vi "Get Calproc.vi"(7 "제목":refnum<vi>, 8 "에러 입력":errorcluster caption="에러 입력(에러 없음)", 11 "Func_ext":string) -> (0 "에러 출력":errorcluster, 1 "Condition":string[][](array[string]), 3 "Func_ext Out":string, 6 "클러스터":T1)   [LabVIEW 2020]
uses:
  Controls/Clst_Get Calproc.ctl
  Controls/Cmd_Read Query.ctl
  Controls/Clst_Query Info.ctl
  Controls/Cmd_File path.ctl
  Controls/Cmd_File Type.ctl
  Variables/Global_Cal Info.vi
  Public/Polymorph/Data Class_2D Str.vi
  Public/Polymorph/Rmv Empt Arr_2D Str.vi
  <vilib>/Utility/file.llb/Read Delimited Spreadsheet (string).vi
  Public/Polymorph/Array Dedup_2D Str.vi
  <vilib>/addons/database/NI_Database_API.lvlib
panel:
  out "제목":string
  out "Data 2":string[][](array[string])
  out "Data":string[][](array[string])
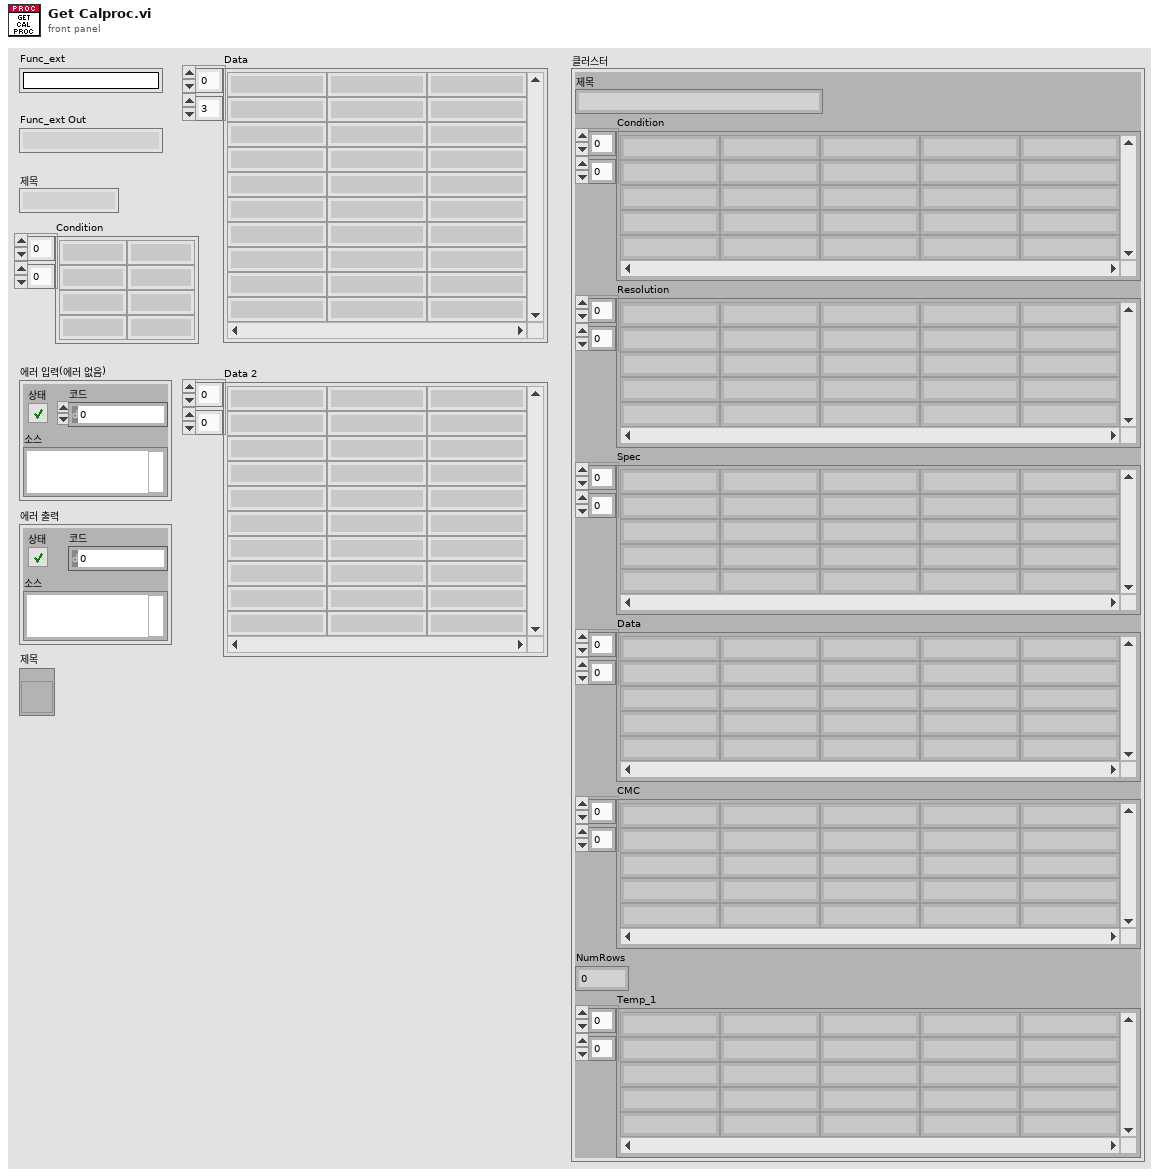
[diagram p1: front panel]
types:
  T1 = typedef "Clst_Get Calproc.ctl" = cluster{"제목":string, "Condition":string[][], "Resolution":string[][], "Spec":string[][], "Data":string[][], "CMC":string[][], "NumRows":u32, "Temp_1":string[][]}
  T2 = typedef "Cmd_Read Query.ctl" = enum16{"교정자 이름 얻기", "인증교정자 얻기", "기술책임자 얻기", "기책부책 얻기", "등록번호 얻기", "등록정보 얻기", "업체정보 얻기", "교정일자(CAMAS) 얻기", "교정일자(CALSTD) 얻기", "교정환경 얻기", "교정절차서 목록 얻기", "교정절차서명 얻기", "교정절차 목록얻기", "교정절차 얻기", "PROC 교정절차 얻기", "PROC SPEC 얻기", "교정절차(Func별) 얻기", "교정절차(Func_ext별) 얻기", "기관코드 얻기", "교정기능(세부분류) 얻기", "교정기능(모델) 얻기", "교정기능 목록 얻기", "교정기능 명칭 얻기", "교정기능 항목명칭 얻기", "DB (사용기준기) 얻기", "DB (기준기이름) 얻기", "DB (기준기이름목록) 얻기", "DB (기준기목록) 얻기", "DB (기준기값) 얻기", "DB (CMC) 얻기", "DB (FUNC) 얻기", "DB (CALNAME) 얻기", "DB (STDNAME) 얻기", "DB (SPEC) 얻기", "모델(항목전체) 얻기", "모델(최대범위) 얻기", "모델(최소범위) 얻기", "모델(최대최소) 얻기", "모델(범위조건) 얻기", "모델(등록요청) 얻기", "모델(형식별) 얻기", "모델(조건별) 얻기", "모델(모델검색) 얻기", "세부분류 목록 얻기", "기준기등록리스트 얻기", "STD Cal Date Check", "DB등록일자 얻기", "적용항목 얻기", "기타정보 얻기", "기준기요청 얻기", "서버버전 얻기"}
  T3 = typedef "Clst_Query Info.ctl" = cluster{"사번":string, "등록번호":string, "업체명":string, "세부분류코드":string, "형식":string, "기기번호":string, "FUNC":string, "FUNC_EXT":string, "옵션":string, "추가문자열":string, "일자":string, "배열 1":string[], "배열 2":string[], "항목명":string, "문자열":string, "이름":string}
  T4 = cluster{"세부분류코드":string, "형식":string, "옵션":string, "측정기명":string, "EXCEL파일명":string, "TEMP":string}
  T5 = typedef "NI_Database_API.lvlib/Conn ObjectReference.ctl" = refnum<k1>
  T6 = typedef "Cmd_File Type.ctl" = enum16{"엑셀", "엑셀(2003)", "텍스트", "설정", "2진", "VI", "CSV", "LOG", "폴더"}
  T7 = typedef "Cmd_File path.ctl" = enum16{"에러로그", "데이터파일경로", "성적서원본", "지난성적서", "Data Files", "경로생성", "Updater", "Template", "설정파일경로", "FTP Upload", "Update 경로", "어플리케이션"}
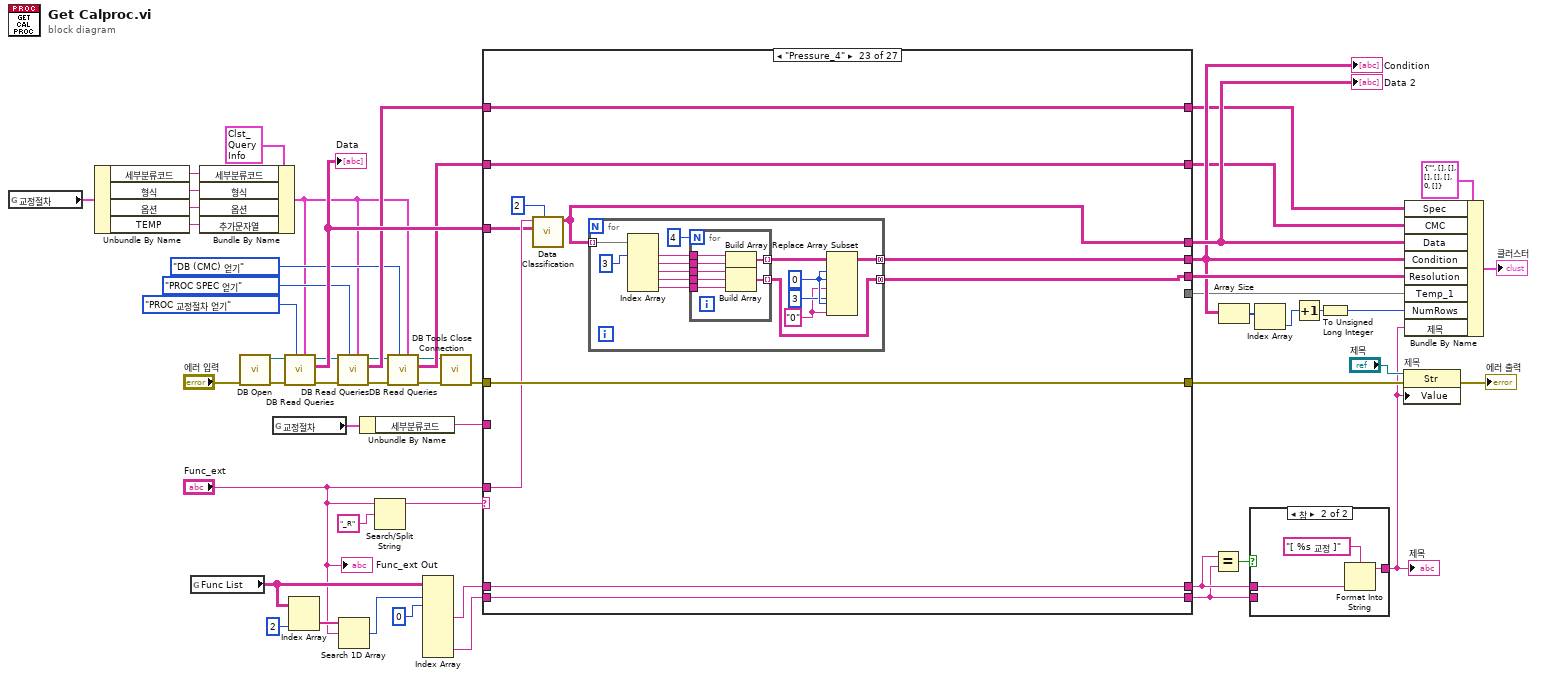
[diagram p0: block diagram]
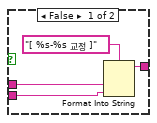
[diagram p2: hidden frame]
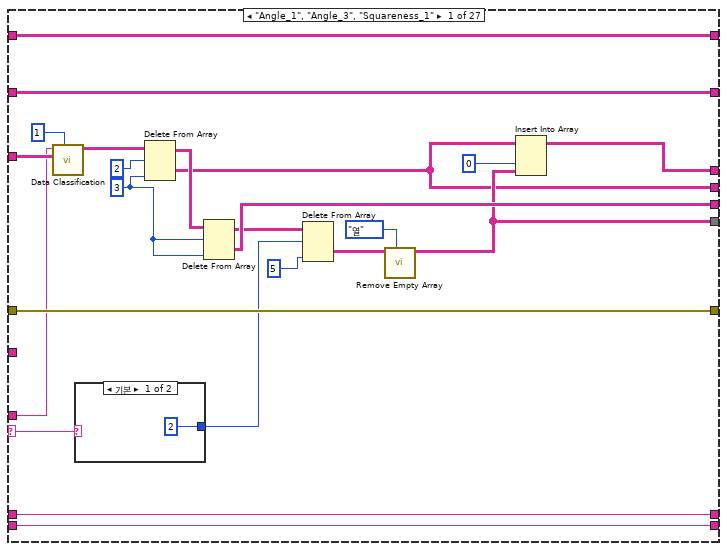
[diagram p3: hidden frame]
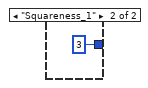
[diagram p4: hidden frame]
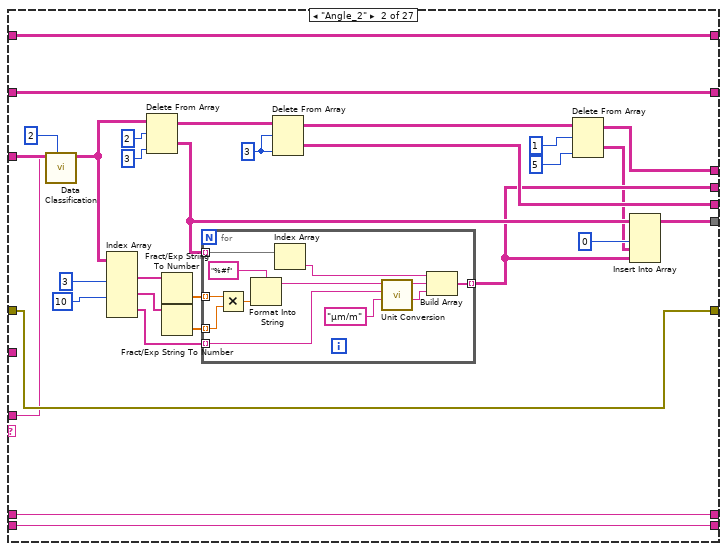
[diagram p5: hidden frame]
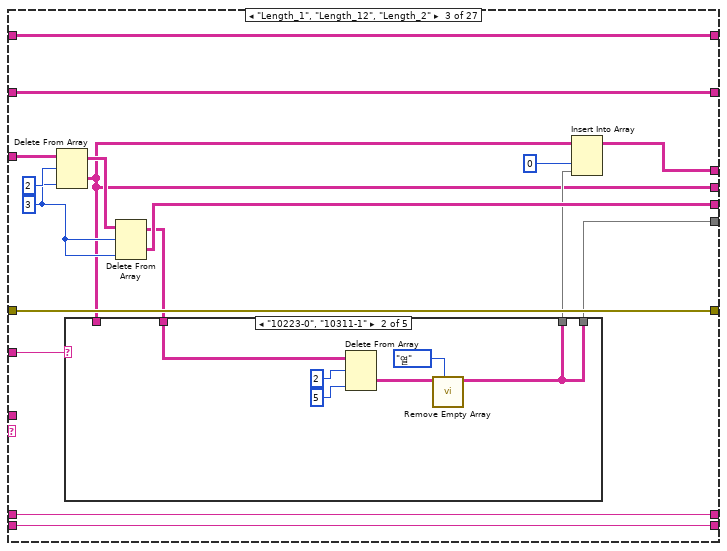
[diagram p6: hidden frame]
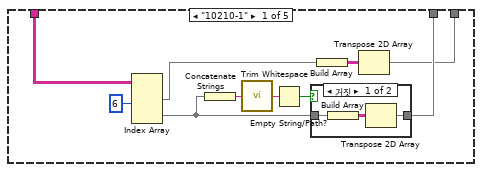
[diagram p7: hidden frame]
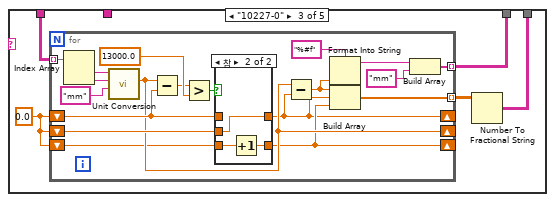
[diagram p9: hidden frame]
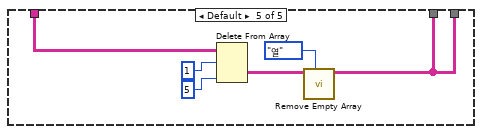
[diagram p12: hidden frame]
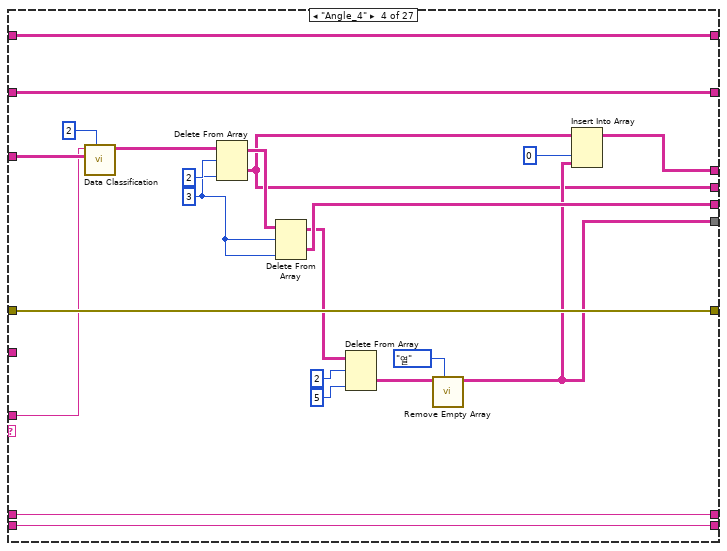
[diagram p13: hidden frame]
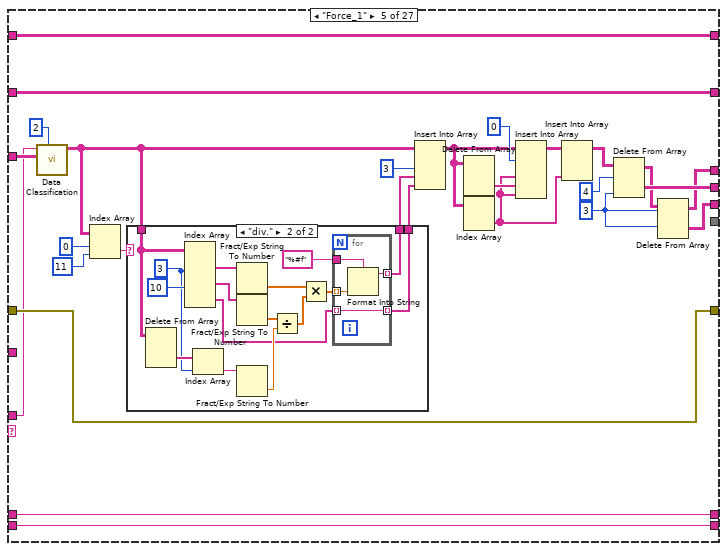
[diagram p14: hidden frame]
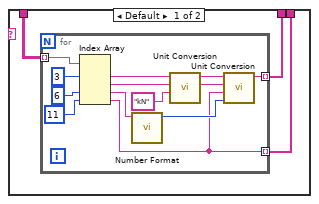
[diagram p15: hidden frame]
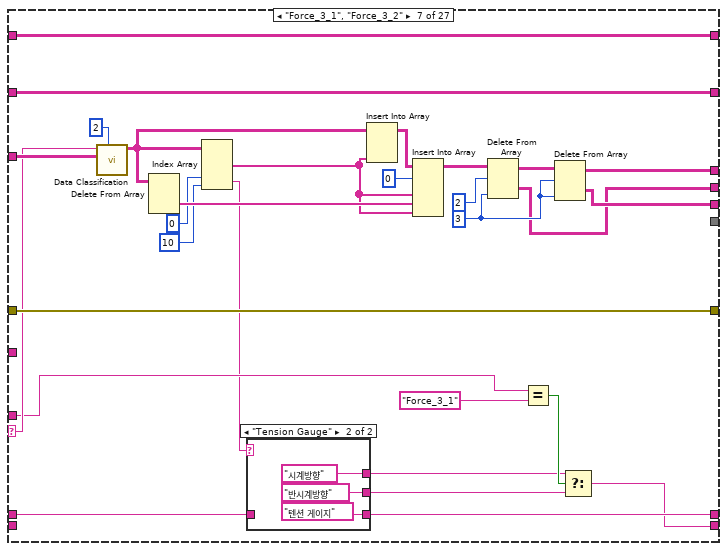
[diagram p17: hidden frame]
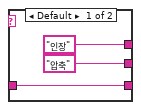
[diagram p18: hidden frame]
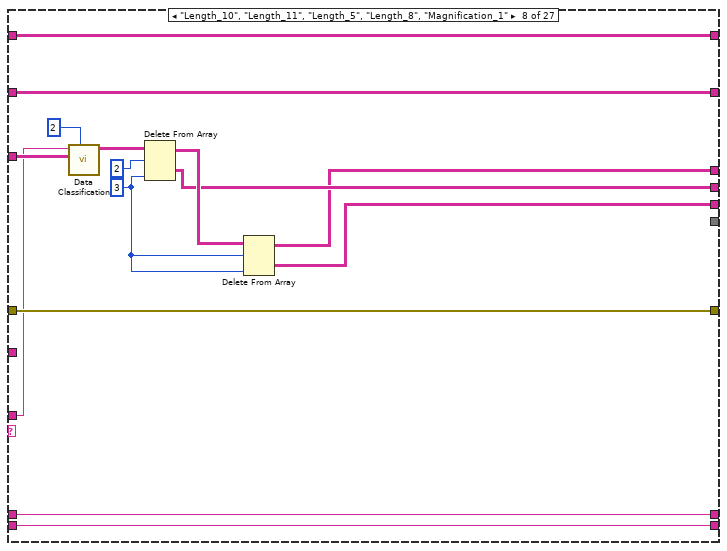
[diagram p19: hidden frame]
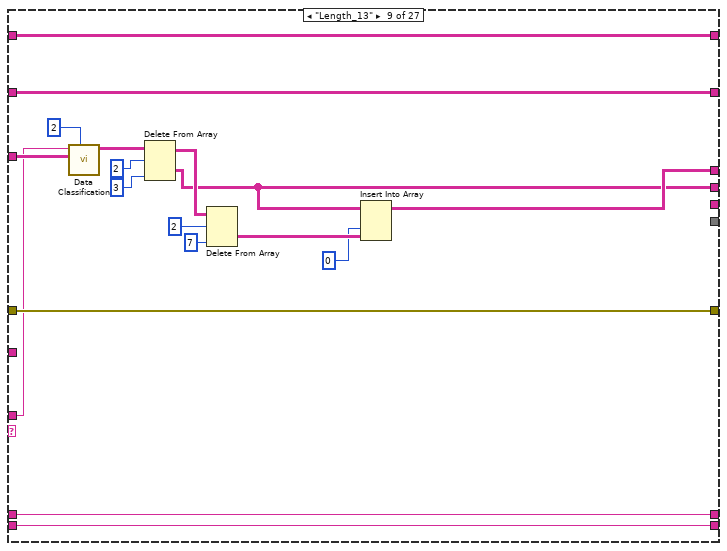
[diagram p20: hidden frame]
diagram:
  n1 = global read "Global_Cal Info.vi" "교정절차"() -> (w29:T4)
  n2 = Unbundle By Name(w29) -> ("세부분류코드"=w28:string, "형식"=w27:string, "옵션"=w26:string, "TEMP"=w13:string)
  n3 = global read "Global_Cal Info.vi" "Func List"() -> (w39:string[][])
  n4 = Bundle By Name(cluster=T3 {"사번"="", "등록번호"="", "업체명"="", "세부분류코드"="", "형식"="", "기기번호"="", "FUNC"="", "FUNC_EXT"="", "옵션"="", "추가문자열"="", "일자"="", "배열 1"=[], "배열 2"=[], "항목명"="", "문자열"="", "이름"=""} ("Query info"), "세부분류코드"=w28, "형식"=w27, "옵션"=w26, "추가문자열"=w13) -> (w15:T3)
  n5 = call "DB Open.vi"("에러 입력"="에러 입력") -> ("에러 출력"=w32:errorcluster, "참조 번호 출력"=w33:T5)  [unwired: 9 in]
  n6 = global read "Global_Cal Info.vi" "교정절차"() -> (w9:T4)
  n7 = call "DB Read Queries.vi"("Query info"=w15, "Query Command"=Cmd_Read_Query."PROC 교정절차 얻기", "에러 입력(에러 없음)"=w32, "참조 번호 입력"=w33) -> ("에러 출력"=w24:errorcluster, "Data"=w31:string[][], "참조 번호 출력"=w25:T5)  [unwired: 3 in, 2 out]
  "Data" <- w31
  n8 = Index Array(array=w39, index (col)=2 ("비활성화된 인덱스 (열)")) -> (element=w37:string[])  [unwired: 1 in]
  n9 = call "DB Read Queries.vi"("Query info"=w15, "Query Command"=Cmd_Read_Query."PROC SPEC 얻기", "에러 입력(에러 없음)"=w24, "참조 번호 입력"=w25) -> ("에러 출력"=w21:errorcluster, "Data"=w23:string[][], "참조 번호 출력"=w20:T5)  [unwired: 3 in, 2 out]
  n10 = Search 1D Array(1D array=w37, element="Func_ext") -> (index of element=w36:i32)  [unwired: 1 in]
  n11 = Unbundle By Name(w9) -> ("세부분류코드"=w8:string)
  n12 = Search/Split String(string="Func_ext", search string/char (-)="_R" ("검색 문자열/문자 (-)")) -> (substring before match=w11:string)  [unwired: 1 in, 2 out]
  n13 = call "DB Read Queries.vi"("Query info"=w15, "Query Command"=Cmd_Read_Query."DB (CMC) 얻기", "에러 입력(에러 없음)"=w21, "참조 번호 입력"=w20) -> ("에러 출력"=w16:errorcluster, "Data"=w18:string[][], "참조 번호 출력"=w17:T5)  [unwired: 3 in, 2 out]
  n14 = Index Array(array=w39, index (row) #1=w36, index (col) #1=0 ("비활성화된 인덱스 (열)")) -> (element #2=w41:string, element #4=w40:string)  [unwired: 6 in, 2 out]
  n15 = call <vilib>:"DB Tools Close Connection.vi"("error in (no error)"=w16, "connection reference"=w17) -> ("error out"=w54:errorcluster)  [unwired: 5 in]
  n16 = case shown="\"Pressure_4\"" w11 {
    selector: w11 -> [w56 _ _ _ _ _ w307 _ _ _ _ _ _ _ _ _ _ w535 w560 w586 w621 _ _ _ w754 w785 _]
    tunnel: w54 -> [w77 w109 w138 w214 w241 w281 w310 w331 w349 w373 w407 w423 w437 w473 w501 w514 w530 w546 w563 w590 w624 w658 w677 w724 w758 w789 w815]
    tunnel: [w77 w109 w138 w214 w241 w281 w310 w331 w349 w373 w407 w423 w437 w473 w501 w514 w530 w546 w563 w590 w624 w658 w677 w724 w758 w789 w815] -> w6
    tunnel: w31 -> [w59 w85 w134 w195 w217 _ w309 w319 w341 w367 w376 w419 w431 w467 w493 w506 w526 w537 w562 w588 w623 w656 w671 w707 w756 w787 w810]
    tunnel: [w62 w82 w122 w201 w233 _ w295 w323 w334 w355 w387 w417 w428 w466 w496 w509 w521 w539 w551 w582 w612 w645 w669 w710 w745 w774 w804] -> w45
    tunnel: [w64 w92 w128 w205 w230 _ w291 w322 w335 _ w376 w412 w426 w465 w497 w510 w516 w540 w550 w583 w613 w642 w668 w711 w741 w770 w800] -> w49
    tunnel: [w70 w98 w130 w207 w231 _ w302 w324 _ w356 _ _ w433 w463 _ _ w522 w541 _ w589 _ w643 w667 w717 w742 w771 w801] -> w51
    tunnel: w41 -> [w76 w103 w137 w213 w226 _ w284 w330 w348 w372 w403 w416 w436 w472 w500 w513 w529 w538 _ _ _ w657 w676 w723 w757 w788 w813]
    tunnel: w40 -> [w61 w80 w123 w202 w222 w280 _ w321 w343 w366 w406 w422 w425 w462 w483 w504 w515 w531 w557 w581 w618 w636 w675 w709 w737 w769 w812]
    tunnel: [w76 w103 w137 w213 w226 w280 w283 w330 w348 w372 w403 w416 w436 w472 w500 w513 w529 w538 w557 w581 w618 w657 w676 w723 w757 w788 w813] -> w4
    tunnel: w18 -> [w75 w104 w136 w212 w240 w278 w306 w329 w347 w371 w404 w420 w434 w470 w499 w512 w528 w533 w559 w585 w620 w654 w670 w722 w753 w784 w809]
    tunnel: [w75 w104 w136 w212 w240 w278 w306 w329 w347 w371 w404 w420 w434 w470 w499 w512 w528 w533 w559 w585 w620 w654 w670 w722 w753 w784 w809] -> w43
    tunnel: w23 -> [w74 w105 w135 w211 w239 w279 w305 w328 w346 w370 w405 w421 w435 w471 w498 w511 w527 w532 w558 w584 w619 w653 w674 w721 w752 w783 w807]
    tunnel: [w74 w105 w135 w211 w239 w279 w305 w328 w346 w370 w405 w421 w435 w471 w498 w511 w527 w532 w558 w584 w619 w653 w674 w721 w752 w783 w807] -> w42
    tunnel: [w63 w87 w124 w203 _ _ _ _ _ _ w374 w411 w427 w460 _ _ w517 _ _ _ _ _ _ _ _ _ string[][] [] ("DATA 출력")] -> w14
    tunnel: "Func_ext" -> [w57 w83 _ w194 w215 _ w294 w317 w339 w368 _ _ w430 _ w494 w507 _ _ _ _ _ w641 w672 w705 _ _ w808]
    tunnel: w8 -> [_ _ w127 _ _ _ _ _ _ _ _ _ w424 _ _ _ _ _ _ _ _ w637 _ _ _ _ _]
    tunnel: [w61 w80 w123 w202 w222 w280 w282 w321 w343 w366 w406 w422 w425 w462 w483 w504 w515 w531 w557 w581 w618 w636 w675 w709 w737 w769 w812] -> w2
    frame "Angle_1", "Angle_3", "Squareness_1" {
      w71 = 3 ("비활성화된 인덱스 (열)")
      n17 = call-poly "Data Classification.vi"("인덱스"=1, "DATA 입력"=w59, "검색 문자열"=w57) -> ("DATA 출력"=w58:string[][])  [unwired: 4 in, 4 out]
      n18 = case shown="기본" w56 {
        tunnel: [2 ("길이") 3 ("길이")] -> w55
        frame Default {
        }
        frame "Squareness_1" {
        }
      }
      n19 = Delete From Array(array=w58, length=2 ("길이"), index (col)=w71) -> (deleted portion=w62:string[][], array with subset deleted=w72:string[][])  [unwired: 1 in]
      n20 = Delete From Array(array=w72, length=w71, index (col)=w71) -> (deleted portion=w70:string[][], array with subset deleted=w69:string[][])  [unwired: 1 in]
      n21 = Delete From Array(array=w69, length=w55, index (col)=5 ("비활성화된 인덱스 (열)")) -> (deleted portion=w67:string[][])  [unwired: 1 in, 1 out]
      n22 = call-poly "Remove Empty Array.vi"("조건"=enum16{"행", "열", "행,열"}."열", "Data in"=w67) -> ("Data out"=w63:string[][])  [unwired: 8 in, 1 out]
      n23 = Insert Into Array(array=w62, index (col)=0 ("비활성화된 인덱스 (열)"), new element=w63) -> (w64:string[][])  [unwired: 1 in]
    }
    frame "Angle_2" {
      w102 = 3 ("비활성화된 인덱스 (열)")
      n24 = call-poly "Data Classification.vi"("인덱스"=2, "DATA 입력"=w85, "검색 문자열"=w83) -> ("DATA 출력"=w84:string[][])  [unwired: 4 in, 4 out]
      n25 = Index Array(array=w84, index (col) #1=3 ("비활성화된 인덱스 (열)"), index (col) #2=10 ("인덱스 (열)")) -> (element #1=w100:string[], element #2=w97:string[], element #3=w95:string[])  [unwired: 4 in]
      n26 = Delete From Array(array=w84, length=2 ("길이"), index (col)=3 ("비활성화된 인덱스 (열)")) -> (deleted portion=w89:string[][], array with subset deleted=w106:string[][])  [unwired: 1 in]
      n27 = Fract/Exp String To Number(string=w100) -> (number=w99:dbl[])  [unwired: 3 in, 1 out]
      n28 = Fract/Exp String To Number(string=w97) -> (number=w96:dbl[])  [unwired: 3 in, 1 out]
      n29 = for {
        tunnel: w89 -> [w117] mode=indexing
        tunnel: w99 -> [w121] mode=indexing
        tunnel: [w116] -> w82 mode=indexing
        tunnel: w96 -> [w120] mode=indexing
        tunnel: w95 -> [w113] mode=indexing
        n30 = Multiply(x=w121, y=w120) -> (x*y=w119:dbl)
        n31 = Format Into String(format string="%#f" ("포맷 문자열"), w119) -> (resulting string=w114:string)  [unwired: 2 in, 1 out]
        n32 = Index Array(array=w117) -> (element=w115:string)  [unwired: 1 in]
        n33 = call "Unit Conversion.vi"("환산단위"="μm/m", "입력단위"=w113, "입력값"=w114) -> ("환산단위"=w110:string, "환산값 (string)"=w111:string)  [unwired: 3 in, 4 out]
        n34 = Build Array(w115, w111, w110) -> (w116:string[])
      }
      n35 = Delete From Array(array=w106, length=w102, index (col)=w102) -> (deleted portion=w98:string[][], array with subset deleted=w93:string[][])  [unwired: 1 in]
      n36 = Delete From Array(array=w93, length=1 ("길이"), index (col)=5 ("비활성화된 인덱스 (열)")) -> (deleted portion=w81:string[][], array with subset deleted=w92:string[][])  [unwired: 1 in]
      n37 = Insert Into Array(array=w89, index (col)=0 ("비활성화된 인덱스 (열)"), new element #1=w81, new element #2=w82) -> (w87:string[][])  [unwired: 1 in]
    }
    frame "Length_1", "Length_12", "Length_2" {
      w131 = 3 ("비활성화된 인덱스 (열)")
      n38 = Delete From Array(array=w134, length=2 ("길이"), index (col)=w131) -> (deleted portion=w122:string[][], array with subset deleted=w132:string[][])  [unwired: 1 in]
      n39 = Delete From Array(array=w132, length=w131, index (col)=w131) -> (deleted portion=w130:string[][], array with subset deleted=w125:string[][])  [unwired: 1 in]
      n40 = case shown="\"10223-0\", \"10311-1\"" w127 {
        tunnel: [w145 w152 w158 _ w187] -> w126
        tunnel: w125 -> [w144 w156 _ _ w191]
        tunnel: [w139 w152 w159 _ w187] -> w124
        tunnel: w122 -> [_ _ w160 _ _]
        frame "10210-1" {
          n41 = Index Array(array=w144, index (col) #1=6 ("비활성화된 인덱스 (열)")) -> (element #1=w141:string[], element #2=w142:string[])  [unwired: 3 in]
          n42 = Concatenate Strings(w142) -> (w148:string)
          n43 = call <vilib>:"Trim Whitespace.vi"("string"=w148) -> ("trimmed string"=w147:string)  [unwired: 1 in]
          n44 = Empty String/Path?(string/path=w147) -> (empty?=w146:bool)
          n45 = case shown="거짓" w146 {
            tunnel: [w150 _] -> w145
            tunnel: w142 -> [w149 _]
            frame False {
              n46 = Build Array(w149) -> (w151:string[][])
              n47 = Transpose 2D Array(2D array=w151) -> (transposed array=w150:string[][])
            }
            frame True {
            }
          }
          n48 = Build Array(w141) -> (w140:string[][])
          n49 = Transpose 2D Array(2D array=w140) -> (transposed array=w139:string[][])
        }
        frame "10223-0", "10311-1" {
          n50 = Delete From Array(array=w156, length=2 ("길이"), index (col)=5 ("비활성화된 인덱스 (열)")) -> (deleted portion=w153:string[][])  [unwired: 1 in, 1 out]
          n51 = call-poly "Remove Empty Array.vi"("조건"=enum16{"행", "열", "행,열"}."열", "Data in"=w153) -> ("Data out"=w152:string[][])  [unwired: 8 in, 1 out]
        }
        frame "10227-0" {
          w161 = 0.0 ("문자열")
          n52 = for {
            shift-right: [w169] -> _
            shift-left: w161 -> [w175]
            tunnel: w160 -> [w176] mode=indexing
            tunnel: [w168] -> w162 mode=indexing
            shift-right: [w172] -> _
            shift-left: w161 -> [w173]
            shift-right: [w170] -> _
            shift-left: w161 -> [w171]
            tunnel: [w163] -> w158 mode=indexing
            n53 = Index Array(array=w176) -> (element #1=w181:string, element #2=w180:string)  [unwired: 2 in]
            n54 = call "Unit Conversion.vi"("환산단위"="mm", "입력단위"=w180, "입력값"=w181) -> ("환산값 (DBL)"=w172:dbl)  [unwired: 3 in, 5 out]
            n55 = Subtract(x=w172, y=w175) -> (x-y=w174:dbl)
            n56 = Greater?(x=w174, y=13000.0) -> (0:w177:bool)
            n57 = case shown="참" w177 {
              tunnel: w175 -> [w183 _]
              tunnel: [w183 w186] -> w169
              tunnel: w173 -> [_ w186]
              tunnel: w171 -> [w182 w185]
              tunnel: [w182 w184] -> w170
              frame False {
              }
              frame True {
                n58 = Increment(x=w185) -> (x+1=w184:dbl)
              }
            }
            n59 = Subtract(x=w172, y=w169) -> (x-y=w167:dbl)
            n60 = Format Into String(format string="%#f" ("포맷 문자열"), w167) -> (resulting string=w165:string)  [unwired: 2 in, 1 out]
            n61 = Build Array(w167, w169, w170) -> (w168:dbl[])
            n62 = Build Array(w165, "mm" ("원소")) -> (w163:string[])
          }
          n63 = Number To Fractional String(number=w162) -> (F-format string=w159:string[][])  [unwired: 3 in]
        }
        frame "10512-0", "10604-2", "10612-1", "10612-2" {
        }
        frame Default {
          n64 = Delete From Array(array=w191, length=1 ("길이"), index (col)=5 ("비활성화된 인덱스 (열)")) -> (deleted portion=w188:string[][])  [unwired: 1 in, 1 out]
          n65 = call-poly "Remove Empty Array.vi"("조건"=enum16{"행", "열", "행,열"}."열", "Data in"=w188) -> ("Data out"=w187:string[][])  [unwired: 8 in, 1 out]
        }
      }
      n66 = Insert Into Array(array=w122, index (col)=0 ("비활성화된 인덱스 (열)"), new element=w126) -> (w128:string[][])  [unwired: 1 in]
    }
    frame "Angle_4" {
      w208 = 3 ("비활성화된 인덱스 (열)")
      n67 = call-poly "Data Classification.vi"("인덱스"=2, "DATA 입력"=w195, "검색 문자열"=w194) -> ("DATA 출력"=w193:string[][])  [unwired: 4 in, 4 out]
      n68 = Delete From Array(array=w193, length=2 ("길이"), index (col)=w208) -> (deleted portion=w201:string[][], array with subset deleted=w209:string[][])  [unwired: 1 in]
      n69 = Delete From Array(array=w209, length=w208, index (col)=w208) -> (deleted portion=w207:string[][], array with subset deleted=w204:string[][])  [unwired: 1 in]
      n70 = Delete From Array(array=w204, length=2 ("길이"), index (col)=5 ("비활성화된 인덱스 (열)")) -> (deleted portion=w197:string[][])  [unwired: 1 in, 1 out]
      n71 = call-poly "Remove Empty Array.vi"("조건"=enum16{"행", "열", "행,열"}."열", "Data in"=w197) -> ("Data out"=w203:string[][])  [unwired: 8 in, 1 out]
      n72 = Insert Into Array(array=w201, index (col)=0 ("비활성화된 인덱스 (열)"), new element=w203) -> (w205:string[][])  [unwired: 1 in]
    }
    frame "Force_1" {
      w221 = 3 ("길이")
      n73 = call-poly "Data Classification.vi"("인덱스"=2, "DATA 입력"=w217, "검색 문자열"=w215) -> ("DATA 출력"=w216:string[][])  [unwired: 4 in, 4 out]
      n74 = Index Array(array=w216, index (row)=0 ("인덱스 (행)"), index (col)=11 ("비활성화된 인덱스 (열)")) -> (element=w223:string)
      n75 = case shown="\"div.\"" w223 {
        tunnel: [w244 w264] -> w237
        tunnel: w216 -> [w242 w263]
        tunnel: [w243 w259] -> w220
        frame Default {
          n76 = for {
            tunnel: [w256] -> w244 mode=indexing
            tunnel: [w245] -> w243 mode=indexing
            tunnel: w242 -> [w252] mode=indexing
            n77 = Index Array(array=w252, index #1=3 ("비활성화된 인덱스 (열)"), index #3=6 ("인덱스 (열)"), index #4=11 ("인덱스 (열)")) -> (element #1=w248:string, element #2=w247:string, element #3=w246:string, element #4=w245:string)  [unwired: 1 in]
            n78 = call "Number Format.vi"("입력값"=w246) -> ("정밀도(단위적용)"=w253:i32)  [unwired: 10 in]
            n79 = call "Unit Conversion.vi"("환산단위"="kN", "입력단위"=w247, "입력값"=w248) -> ("환산단위"=w254:string, "환산값 (string)"=w257:string)  [unwired: 3 in, 4 out]
            n80 = call "Unit Conversion.vi"("소수점 자리수"=w253, "환산단위"=w245, "입력단위"=w254, "입력값"=w257) -> ("환산값 (string)"=w256:string)  [unwired: 2 in, 5 out]
          }
        }
        frame "div." {
          w262 = 3 ("인덱스 (열)")
          n81 = Delete From Array(array=w263) -> (deleted portion=w271:string[])  [unwired: 3 in, 1 out]
          n82 = Index Array(array=w263, index (col) #1=w262, index (col) #2=10 ("비활성화된 인덱스 (열)")) -> (element #1=w261:string[], element #2=w272:string[], element #3=w258:string[])  [unwired: 4 in]
          n83 = Index Array(array=w271, index=w262) -> (element=w270:string)
          n84 = Fract/Exp String To Number(string=w261) -> (number=w266:dbl[])  [unwired: 3 in, 1 out]
          n85 = Fract/Exp String To Number(string=w272) -> (number=w269:dbl[])  [unwired: 3 in, 1 out]
          n86 = Fract/Exp String To Number(string=w270) -> (number=w268:dbl)  [unwired: 3 in, 1 out]
          n87 = Divide(x=w269, y=w268) -> (x/y=w267:dbl[])
          n88 = Multiply(x=w266, y=w267) -> (x*y=w265:dbl[])
          n89 = for {
            tunnel: w265 -> [w277] mode=indexing
            tunnel: [w276] -> w264 mode=indexing
            tunnel: "%#f" ("포맷 문자열") -> [w275]
            tunnel: [w274] -> w259 mode=indexing
            tunnel: w258 -> [w274] mode=indexing
            n90 = Format Into String(format string=w275, w277) -> (resulting string=w276:string)  [unwired: 2 in, 1 out]
          }
        }
      }
      n91 = Insert Into Array(array=w216, index (col)=3 ("비활성화된 인덱스 (열)"), new element #1=w237, new element #2=w220) -> (w234:string[][])  [unwired: 1 in]
      n92 = Delete From Array(array=w234) -> (deleted portion=w235:string[])  [unwired: 3 in, 1 out]
      n93 = Index Array(array=w234) -> (element=w227:string[])  [unwired: 2 in]
      n94 = Insert Into Array(array=w234, index (row)=0 ("인덱스 (행)"), new element #1=w227, new element #2=w235, new element #3=w227) -> (w229:string[][])  [unwired: 1 in]
      n95 = Insert Into Array(array=w229, new element=w227) -> (w228:string[][])  [unwired: 2 in]
      n96 = Delete From Array(array=w228, length=4 ("길이"), index (col)=w221) -> (deleted portion=w233:string[][], array with subset deleted=w232:string[][])  [unwired: 1 in]
      n97 = Delete From Array(array=w232, length=w221, index (col)=w221) -> (deleted portion=w231:string[][], array with subset deleted=w230:string[][])  [unwired: 1 in]
    }
    frame "Force_2" {
    }
    frame "Force_3_1", "Force_3_2" {
      w301 = 3 ("비활성화된 인덱스 (열)")
      n98 = call-poly "Data Classification.vi"("인덱스"=2, "DATA 입력"=w309, "검색 문자열"=w307) -> ("DATA 출력"=w290:string[][])  [unwired: 4 in, 4 out]
      n99 = Delete From Array(array=w290) -> (deleted portion=w299:string[])  [unwired: 3 in, 1 out]
      n100 = Index Array(array=w290, index (row) #2=0 ("인덱스 (행)"), index (col) #2=10 ("비활성화된 인덱스 (열)")) -> (element #1=w297:string[], element #2=w287:string)  [unwired: 2 in]
      n101 = case shown="\"Tension Gauge\"" w287 {
        tunnel: ["인장" "시계방향"] -> w286
        tunnel: ["압축" "반시계방향"] -> w285
        tunnel: w284 -> [w311 _]
        tunnel: [w311 "텐션 게이지" ("문자열")] -> w283
        frame Default {
        }
        frame "Tension Gauge" {
        }
      }
      n102 = Insert Into Array(array=w290, new element=w297) -> (w298:string[][])  [unwired: 2 in]
      n103 = Insert Into Array(array=w298, index (row)=0 ("인덱스 (행)"), new element #1=w297, new element #2=w299, new element #3=w297) -> (w296:string[][])  [unwired: 1 in]
      n104 = Delete From Array(array=w296, length=2 ("길이"), index (col)=w301) -> (deleted portion=w295:string[][], array with subset deleted=w303:string[][])  [unwired: 1 in]
      n105 = Equal?(x=w294, y="Force_3_1") -> (x = y?=w292:bool)
      n106 = Delete From Array(array=w303, length=w301, index (col)=w301) -> (deleted portion=w302:string[][], array with subset deleted=w291:string[][])  [unwired: 1 in]
      n107 = Select(t=w286, s=w292, f=w285) -> (s? t:f=w282:string)
    }
    frame "Length_10", "Length_11", "Length_5", "Length_8", "Magnification_1" {
      w325 = 3 ("비활성화된 인덱스 (열)")
      n108 = call-poly "Data Classification.vi"("인덱스"=2, "DATA 입력"=w319, "검색 문자열"=w317) -> ("DATA 출력"=w318:string[][])  [unwired: 4 in, 4 out]
      n109 = Delete From Array(array=w318, length=2 ("길이"), index (col)=w325) -> (deleted portion=w323:string[][], array with subset deleted=w326:string[][])  [unwired: 1 in]
      n110 = Delete From Array(array=w326, length=w325, index (col)=w325) -> (deleted portion=w324:string[][], array with subset deleted=w322:string[][])  [unwired: 1 in]
    }
    frame "Length_13" {
      n111 = call-poly "Data Classification.vi"("인덱스"=2, "DATA 입력"=w341, "검색 문자열"=w339) -> ("DATA 출력"=w340:string[][])  [unwired: 4 in, 4 out]
      n112 = Delete From Array(array=w340, length=2 ("길이"), index (col)=3 ("비활성화된 인덱스 (열)")) -> (deleted portion=w334:string[][], array with subset deleted=w337:string[][])  [unwired: 1 in]
      n113 = Delete From Array(array=w337, length=2 ("길이"), index (col)=7 ("비활성화된 인덱스 (열)")) -> (deleted portion=w333:string[][])  [unwired: 1 in, 1 out]
      n114 = Insert Into Array(array=w334, index (col)=0 ("비활성화된 인덱스 (열)"), new element=w333) -> (w335:string[][])  [unwired: 1 in]
    }
    frame "Length_14" {
      w351 = string[] [""]
      n115 = call-poly "Data Classification.vi"("인덱스"=2, "DATA 입력"=w367, "검색 문자열"=w368) -> ("DATA 출력"=w365:string[][])  [unwired: 4 in, 4 out]
      n116 = Delete From Array(array=w365, length=2 ("길이"), index (col)=10 ("비활성화된 인덱스 (열)")) -> (deleted portion=w352:string[][], array with subset deleted=w360:string[][])  [unwired: 1 in]
      n117 = Delete From Array(array=w360, length=2 ("길이"), index (col)=3 ("비활성화된 인덱스 (열)")) -> (deleted portion=w350:string[][], array with subset deleted=w357:string[][])  [unwired: 1 in]
      n118 = Delete From Array(array=w357, length=3 ("길이"), index (col)=3 ("비활성화된 인덱스 (열)")) -> (deleted portion=w356:string[][])  [unwired: 1 in, 1 out]
      n119 = Insert Into Array(array=string[][] [["등급"], [""], [""], ["리드각"], [""], [""], ["측정력(N)"], [""], [""], ["F0"], [""], ["L0"], [""], [""]], index (col)=0 ("비활성화된 인덱스 (열)"), new element #1=w351, new element #2=w352, new element #3=w350, new element #4=w351, new element #5=w351) -> (w355:string[][])  [unwired: 1 in]
    }
    frame "Length_15" {
      w394 = "mm" ("환산단위")
      n120 = Delete From Array(array=w376, length=4 ("길이"), index (col)=9 ("비활성화된 인덱스 (열)")) -> (deleted portion=w400:string[][])  [unwired: 1 in, 1 out]
      n121 = Index Array(array=w400) -> (element=w399:string[])  [unwired: 2 in]
      n122 = Index Array(array=w399) -> (element #1=w398:string, element #2=w397:string, element #3=w396:string, element #4=w395:string)  [unwired: 4 in]
      n123 = call "Unit Conversion.vi"("환산단위"=w394, "입력단위"=w397, "입력값"=w398) -> ("환산값 (DBL)"=w386:dbl, "환산값 (string)"=w393:string)  [unwired: 3 in, 4 out]
      n124 = call "Unit Conversion.vi"("환산단위"=w394, "입력단위"=w395, "입력값"=w396) -> ("환산값 (DBL)"=w385:dbl, "환산값 (string)"=w392:string)  [unwired: 3 in, 4 out]
      n125 = Square(x=w386) -> (x^2=w384:dbl)
      n126 = Square(x=w385) -> (x^2=w383:dbl)
      n127 = Add(x=w384, y=w383) -> (x+y=w382:dbl)
      n128 = Square Root(x=w382) -> (sqrt(x)=w381:dbl)
      n129 = Format Into String(format string="%d" ("포맷 문자열"), w381) -> (resulting string=w390:string)  [unwired: 2 in, 1 out]
      n130 = Build Array(w393, w392, w390) -> (w388:string[])
      n131 = for {
        tunnel: string[] ["가로", "세로", "대각선"] -> [w410] mode=indexing
        tunnel: w388 -> [w409] mode=indexing
        tunnel: [w408] -> w387 mode=indexing
        n132 = Build Array(w410, w409) -> (w408:string[])
      }
      n133 = call "Create File Path.vi"("파일타입"=Cmd_File_Type."CSV", "항목"=Cmd_File_path."데이터파일경로", "문자열 in"="Surface Plate") -> ("파일경로"=w375:path)  [unwired: 5 in, 3 out]
      n134 = call-poly <vilib>:"Read Delimited Spreadsheet.vi"("file path (dialog if empty)"=w375, "delimiter (\\t)"="," ("delimiter (\\t)")) -> ("all rows"=w374:string[][])  [unwired: 8 in, 5 out]
    }
    frame "Length_16" {
      w414 = 3 ("비활성화된 인덱스 (열)")
      n135 = Delete From Array(array=w419, length=2 ("길이"), index (col)=w414) -> (deleted portion=w417:string[][], array with subset deleted=w415:string[][])  [unwired: 1 in]
      n136 = Delete From Array(array=w415, length=w414, index (col)=8 ("비활성화된 인덱스 (열)")) -> (deleted portion=w412:string[][], array with subset deleted=w411:string[][])  [unwired: 1 in]
    }
    frame "Length_3" {
      n137 = call-poly "Data Classification.vi"("인덱스"=2, "DATA 입력"=w431, "검색 문자열"=w430) -> ("DATA 출력"=w429:string[][])  [unwired: 4 in, 4 out]
      n138 = case shown="\"10236-0\", 기본" w424 {
        tunnel: [w440 w456] -> w433
        tunnel: w429 -> [w447 w455]
        tunnel: [w445 w450] -> w428
        tunnel: [w438 w449] -> w427
        tunnel: [w444 w448] -> w426
        frame "10517-0" {
          w443 = 3 ("비활성화된 인덱스 (열)")
          n139 = Delete From Array(array=w447, length=2 ("길이"), index (col)=w443) -> (deleted portion=w445:string[][], array with subset deleted=w444:string[][])  [unwired: 1 in]
          n140 = Delete From Array(array=w444, length=w443, index (col)=w443) -> (deleted portion=w440:string[][], array with subset deleted=w439:string[][])  [unwired: 1 in]
          n141 = Delete From Array(array=w439, length=5 ("길이"), index (col)=0 ("비활성화된 인덱스 (열)")) -> (array with subset deleted=w438:string[][])  [unwired: 1 in, 1 out]
        }
        frame "10236-0", Default {
          w457 = 3 ("비활성화된 인덱스 (열)")
          n142 = Delete From Array(array=w455, length=2 ("길이"), index (col)=w457) -> (deleted portion=w450:string[][], array with subset deleted=w458:string[][])  [unwired: 1 in]
          n143 = Delete From Array(array=w458, length=w457, index (col)=w457) -> (deleted portion=w456:string[][], array with subset deleted=w454:string[][])  [unwired: 1 in]
          n144 = Delete From Array(array=w454, index (col)=5 ("비활성화된 인덱스 (열)")) -> (deleted portion=w452:string[], array with subset deleted=w448:string[][])  [unwired: 2 in]
          n145 = Insert Into Array(array=w450, index (col)=0 ("비활성화된 인덱스 (열)"), new element=w452) -> (w449:string[][])  [unwired: 1 in]
        }
      }
    }
    frame "Length_4" {
      w464 = 3 ("비활성화된 인덱스 (열)")
      n146 = Delete From Array(array=w467, length=2 ("길이"), index (col)=w464) -> (deleted portion=w466:string[][], array with subset deleted=w468:string[][])  [unwired: 1 in]
      n147 = Delete From Array(array=w468, length=w464, index (col)=w464) -> (deleted portion=w461:string[][], array with subset deleted=w465:string[][])  [unwired: 1 in]
      n148 = for {
        tunnel: w461 -> [w482] mode=indexing
        tunnel: [w480] -> w463 mode=indexing
        tunnel: [w475] -> w460 mode=indexing
        w477 = "0.00001" ("새 원소/부분배열")
        w474 = "2급" ("새 원소/부분배열")
        n149 = Build Array(w474, w477, w477, "mm" ("새 원소/부분배열")) -> (w475:string[])
        n150 = Replace Array Subset(array=w482, new element #1=w474, index #1=0 ("인덱스"), new element #2="0.01" ("새 원소/부분배열"), index #2=2 ("인덱스")) -> (w480:string[])
      }
    }
    frame "Length_6_1", "Length_6_2" {
      n151 = call-poly "Data Classification.vi"("인덱스"=2, "DATA 입력"=w493, "검색 문자열"=w494) -> ("DATA 출력"=w492:string[][])  [unwired: 4 in, 4 out]
      n152 = Delete From Array(array=w492, length=2 ("길이"), index (col)=3 ("비활성화된 인덱스 (열)")) -> (deleted portion=w484:string[][], array with subset deleted=w490:string[][])  [unwired: 1 in]
      n153 = Delete From Array(array=w490, length=1 ("길이"), index (col)=8 ("비활성화된 인덱스 (열)")) -> (deleted portion=w486:string[][], array with subset deleted=w497:string[][])  [unwired: 1 in]
      n154 = Insert Into Array(array=w486, index (col)=0 ("비활성화된 인덱스 (열)"), new element=w484) -> (w496:string[][])  [unwired: 1 in]
    }
    frame "Length_7" {
      n155 = call-poly "Data Classification.vi"("인덱스"=2, "DATA 입력"=w506, "검색 문자열"=w507) -> ("DATA 출력"=w505:string[][])  [unwired: 4 in, 4 out]
      n156 = Delete From Array(array=w505, length=2 ("길이"), index (col)=3 ("비활성화된 인덱스 (열)")) -> (deleted portion=w509:string[][], array with subset deleted=w510:string[][])  [unwired: 1 in]
    }
    frame "Length_9" {
      w523 = 3 ("비활성화된 인덱스 (열)")
      n157 = Delete From Array(array=w526, length=2 ("길이"), index (col)=w523) -> (deleted portion=w521:string[][], array with subset deleted=w524:string[][])  [unwired: 1 in]
      n158 = Delete From Array(array=w524, length=w523, index (col)=w523) -> (deleted portion=w522:string[][], array with subset deleted=w520:string[][])  [unwired: 1 in]
      n159 = Delete From Array(array=w520, length=3 ("길이"), index (col)=4 ("비활성화된 인덱스 (열)")) -> (deleted portion=w517:string[][], array with subset deleted=w516:string[][])  [unwired: 1 in]
    }
    frame "Mass_1_1", "Mass_1_2", "Mass_1_3" {
      w543 = 3 ("비활성화된 인덱스 (열)")
      n160 = call-poly "Data Classification.vi"("인덱스"=2, "DATA 입력"=w537, "검색 문자열"=w535) -> ("DATA 출력"=w534:string[][])  [unwired: 4 in, 4 out]
      n161 = Delete From Array(array=w534, length=2 ("길이"), index (col)=w543) -> (deleted portion=w539:string[][], array with subset deleted=w544:string[][])  [unwired: 1 in]
      n162 = Delete From Array(array=w544, length=3 ("길이"), index (col)=w543) -> (deleted portion=w541:string[][], array with subset deleted=w540:string[][])  [unwired: 1 in]
    }
    frame "Mass_2_1" {
      n163 = call-poly "Data Classification.vi"("인덱스"=2, "DATA 입력"=w562, "검색 문자열"=w560) -> ("DATA 출력"=w554:string[][])  [unwired: 4 in, 4 out]
      n164 = Delete From Array(array=w554, length=2 ("길이"), index (col)=3 ("비활성화된 인덱스 (열)")) -> (deleted portion=w549:string[][], array with subset deleted=w553:string[][])  [unwired: 1 in]
      n165 = Delete From Array(array=w553, index (col)=7 ("비활성화된 인덱스 (열)")) -> (deleted portion=w547:string[], array with subset deleted=w550:string[][])  [unwired: 2 in]
      n166 = Index Array(array=w547) -> (element=w548:string)  [unwired: 1 in]
      n167 = case shown="기본" w548 {
        tunnel: w549 -> [_ w566]
        tunnel: w547 -> [_ w565]
        tunnel: [_ w564] -> w551
        frame "설정" {
        }
        frame Default {
          n168 = for {
            tunnel: w566 -> [w576] mode=indexing
            tunnel: w565 -> [w570] mode=indexing
            tunnel: [w571] -> w564 mode=indexing
            n169 = Index Array(array=w576) -> (element #1=w568:string, element #2=w575:string)  [unwired: 2 in]
            n170 = call "Unit Conversion.vi"("환산단위"="g", "입력단위"=w575, "입력값"=w568) -> ("입력단위"=w567:string, "환산단위"=w572:string, "환산값 (string)"=w573:string)  [unwired: 3 in, 3 out]
            n171 = Build Array(w570, "", w568, w567, w573, w572) -> (w571:string[])
          }
        }
      }
    }
    frame "Mass_2_1_old" {
      n172 = call-poly "Data Classification.vi"("인덱스"=2, "DATA 입력"=w588, "검색 문자열"=w586) -> ("DATA 출력"=w580:string[][])  [unwired: 4 in, 4 out]
      n173 = Index Array(array=w580, index (row)=0 ("인덱스 (행)"), index (col)=9 ("비활성화된 인덱스 (열)")) -> (element=w577:string)
      n174 = case shown="기본" w577 {
        tunnel: [_ w600] -> w589
        tunnel: [_ w596] -> w583
        tunnel: [_ w591] -> w582
        tunnel: w580 -> [_ w593]
        frame "설정" {
        }
        frame Default {
          w602 = 3 ("비활성화된 인덱스 (열)")
          n175 = Delete From Array(array=w593, length=2 ("길이"), index (col)=w602) -> (deleted portion=w599:string[][], array with subset deleted=w603:string[][])  [unwired: 1 in]
          n176 = Delete From Array(array=w603, length=3 ("길이"), index (col)=w602) -> (deleted portion=w600:string[][], array with subset deleted=w598:string[][])  [unwired: 1 in]
          n177 = Delete From Array(array=w598, index (col)=4 ("비활성화된 인덱스 (열)")) -> (deleted portion=w595:string[], array with subset deleted=w596:string[][])  [unwired: 2 in]
          n178 = Insert Into Array(array=w599, index (col)=0 ("비활성화된 인덱스 (열)"), new element=w595) -> (w592:string[][])  [unwired: 1 in]
          n179 = for {
            tunnel: w592 -> [w608] mode=indexing
            tunnel: [w606] -> w591 mode=indexing
            n180 = Index Array(array=w608) -> (element #2=w611:string, element #3=w610:string)  [unwired: 3 in, 1 out]
            n181 = call "Unit Conversion.vi"("환산단위"="g", "입력단위"=w610, "입력값"=w611) -> ("환산단위"=w605:string, "환산값 (string)"=w607:string)  [unwired: 3 in, 4 out]
            n182 = Insert Into Array(array=w608, new element #1=w607, new element #2=w605) -> (w606:string[])  [unwired: 1 in]
          }
        }
      }
    }
    frame "Mass_2_2" {
      n183 = call-poly "Data Classification.vi"("인덱스"=2, "DATA 입력"=w623, "검색 문자열"=w621) -> ("DATA 출력"=w617:string[][])  [unwired: 4 in, 4 out]
      n184 = Index Array(array=w617, index (row)=0 ("인덱스 (행)"), index (col)=9 ("비활성화된 인덱스 (열)")) -> (element=w614:string)
      n185 = case shown="기본" w614 {
        tunnel: w617 -> [_ w635]
        tunnel: [_ w625] -> w613
        tunnel: [_ w627] -> w612
        frame "설정" {
        }
        frame Default {
          n186 = Delete From Array(array=w635, length=4 ("길이"), index (col)=9 ("비활성화된 인덱스 (열)")) -> (deleted portion=w629:string[][], array with subset deleted=w632:string[][])  [unwired: 1 in]
          n187 = Delete From Array(array=w632, length=2 ("길이"), index (col)=3 ("비활성화된 인덱스 (열)")) -> (deleted portion=w628:string[][], array with subset deleted=w625:string[][])  [unwired: 1 in]
          n188 = Insert Into Array(array=w629, index (col)=4 ("비활성화된 인덱스 (열)"), new element=w628) -> (w627:string[][])  [unwired: 1 in]
        }
      }
    }
    frame "Pressure_1", "Pressure_2", "Pressure_3" {
      n189 = call-poly "Data Classification.vi"("인덱스"=2, "DATA 입력"=w656, "검색 문자열"=w641) -> ("DATA 출력"=w649:string[][])  [unwired: 4 in, 4 out]
      n190 = Array Size(array=w649) -> (size(s)=w652:i32[])
      n191 = Index Array(array=w652) -> (element #2=w651:i32)  [unwired: 2 in, 1 out]
      n192 = for {
        N: w651 -> [_]
        tunnel: w649 -> [w666]
        tunnel: [w663] -> w650 mode=indexing
        i -> [w665]
        n193 = Index Array(array=w666, index (col)=w665) -> (element=w664:string[])  [unwired: 1 in]
        n194 = Reverse 1D Array(array=w664) -> (reversed array=w663:string[])
      }
      n195 = case shown="기본" w637 {
        tunnel: [w659 11 ("비활성화된 인덱스 (열)")] -> w640
        tunnel: [w659 5 ("길이")] -> w639
        tunnel: [w659 3 ("길이")] -> w638
        frame Default {
          w659 = 3 ("비활성화된 인덱스 (열)")
        }
        frame "20409-0" {
        }
      }
      n196 = Transpose 2D Array(2D array=w650) -> (transposed array=w648:string[][])
      n197 = Insert Into Array(array=w649, new element=w648) -> (w647:string[][])  [unwired: 2 in]
      n198 = Delete From Array(array=w647, length=2 ("길이"), index (col)=w640) -> (deleted portion=w645:string[][], array with subset deleted=w644:string[][])  [unwired: 1 in]
      n199 = Delete From Array(array=w644, length=w638, index (col)=w639) -> (deleted portion=w643:string[][], array with subset deleted=w642:string[][])  [unwired: 1 in]
    }
    frame "Pressure_4" {
      n200 = call-poly "Data Classification.vi"("인덱스"=2, "DATA 입력"=w671, "검색 문자열"=w672) -> ("DATA 출력"=w668:string[][])  [unwired: 4 in, 4 out]
      n201 = for {
        tunnel: w668 -> [w691] mode=indexing
        tunnel: [w681] -> w669 mode=concatenating
        tunnel: [w684] -> w667 mode=concatenating
        w678 = "0"
        w680 = 0 ("인덱스 (행)")
        n202 = Index Array(array=w691, index #1=3 ("인덱스")) -> (element #1=w689:string, element #2=w688:string, element #3=w687:string, element #4=w686:string, element #5=w685:string)  [unwired: 4 in]
        n203 = for {
          N: 4 -> [_]
          tunnel: w689 -> [w698]
          tunnel: w688 -> [w697]
          tunnel: w687 -> [w696]
          tunnel: w686 -> [w695]
          tunnel: w685 -> [w694]
          tunnel: [w693] -> w684 mode=indexing
          tunnel: [w692] -> w682 mode=indexing
          n204 = Build Array(w698, w697) -> (w692:string[])
          n205 = Build Array(w696, w695, w694) -> (w693:string[])
        }
        n206 = Replace Array Subset(array=w682, new element #1=w678, index (row) #1=w680, index (col) #1=w680, new element #2=w678, index (row) #2=3 ("비활성화된 인덱스 (행)"), index (col) #2=w680) -> (w681:string[][])
      }
    }
    frame "Straightness_1" {
      w718 = 3 ("비활성화된 인덱스 (열)")
      n207 = call-poly "Data Classification.vi"("인덱스"=1, "DATA 입력"=w707, "검색 문자열"=w705) -> ("DATA 출력"=w706:string[][])  [unwired: 4 in, 4 out]
      n208 = Delete From Array(array=w706, length=2 ("길이"), index (col)=w718) -> (deleted portion=w710:string[][], array with subset deleted=w719:string[][])  [unwired: 1 in]
      n209 = Delete From Array(array=w719, length=w718, index (col)=w718) -> (deleted portion=w717:string[][], array with subset deleted=w716:string[][])  [unwired: 1 in]
      n210 = Delete From Array(array=w716, length=2 ("길이"), index (col)=5 ("비활성화된 인덱스 (열)")) -> (deleted portion=w714:string[][])  [unwired: 1 in, 1 out]
      n211 = call-poly "Remove Empty Array.vi"("조건"=enum16{"행", "열", "행,열"}."열", "Data in"=w714) -> ("Data out"=w699:string[][])  [unwired: 8 in, 1 out]
      n212 = call-poly "Array Deduplication.vi"("배열 in"=w699) -> ("배열 out"=w703:string[][])  [unwired: 9 in, 1 out]
      n213 = Index Array(array=w699, index (col)=0 ("비활성화된 인덱스 (열)")) -> (element=w702:string[])  [unwired: 1 in]
      n214 = for {
        tunnel: w703 -> [w727] mode=indexing
        tunnel: w702 -> [w726]
        tunnel: [w725] -> w700 mode=concatenating
        n215 = for {
          shift-right: [w732] -> _
          shift-left: -1 ("숫자") -> [w736]
          tunnel: w727 -> [w734]
          tunnel: w726 -> [w729] mode=indexing
          tunnel: [w731] -> w725 mode=indexing if=w730
          n216 = Concatenate Strings(w734) -> (w733:string)
          n217 = Increment(x=w736) -> (x+1=w735:i32)
          n218 = Equal?(x=w733, y=w729) -> (x = y?=w730:bool)
          n219 = Select(t=w735, s=w730, f=w736) -> (s? t:f=w732:i32)
          n220 = Number To Decimal String(number=w732) -> (decimal integer string=w731:string)  [unwired: 1 in]
        }
      }
      n221 = Insert Into Array(array=w710, index (col)=0 ("비활성화된 인덱스 (열)"), new element #1=w699, new element #2=w700) -> (w711:string[][])  [unwired: 1 in]
    }
    frame "Torque_1" {
      w743 = 3 ("비활성화된 인덱스 (열)")
      w751 = 0 ("인덱스 (행)")
      n222 = call-poly "Data Classification.vi"("인덱스"=2, "DATA 입력"=w756, "검색 문자열"=w754) -> ("DATA 출력"=w749:string[][])  [unwired: 4 in, 4 out]
      n223 = for {
        tunnel: w749 -> [w764] mode=indexing
        tunnel: [w760] -> w748 mode=indexing
        tunnel: [w759] -> w747
        i -> [w759]
        n224 = Index Array(array=w764, index #1=3 ("인덱스")) -> (element #1=w767:string, element #2=w766:string)  [unwired: 1 in]
        n225 = call "Unit Conversion.vi"("환산단위"="N·m", "입력단위"=w766, "입력값"=w767) -> ("환산단위"=w762:string, "환산값 (string)"=w763:string)  [unwired: 3 in, 4 out]
        n226 = Insert Into Array(array=w764, index=5 ("인덱스"), new element #1=w763, new element #2=w762) -> (w760:string[])
      }
      n227 = Index Array(array=w748, index (row) #1=w747, index (row) #2=w751) -> (element #1=w750:string[], element #2=w738:string[])  [unwired: 2 in]
      n228 = Insert Into Array(array=w748, index (row)=w751, new element #1=w738, new element #2=w750, new element #3=w738) -> (w740:string[][])  [unwired: 1 in]
      n229 = Insert Into Array(array=w740, new element=w738) -> (w739:string[][])  [unwired: 2 in]
      n230 = Delete From Array(array=w739, length=4 ("길이"), index (col)=w743) -> (deleted portion=w745:string[][], array with subset deleted=w744:string[][])  [unwired: 1 in]
      n231 = Delete From Array(array=w744, length=w743, index (col)=w743) -> (deleted portion=w742:string[][], array with subset deleted=w741:string[][])  [unwired: 1 in]
    }
    frame "Torque_2" {
      w772 = 3 ("비활성화된 인덱스 (열)")
      w782 = 0 ("인덱스 (행)")
      n232 = call-poly "Data Classification.vi"("인덱스"=2, "DATA 입력"=w787, "검색 문자열"=w785) -> ("DATA 출력"=w778:string[][])  [unwired: 4 in, 4 out]
      n233 = for {
        tunnel: w778 -> [w795] mode=indexing
        tunnel: [w791] -> w777 mode=indexing
        tunnel: [w790] -> w776
        i -> [w790]
        n234 = Index Array(array=w795, index #1=3 ("인덱스")) -> (element #1=w798:string, element #2=w797:string)  [unwired: 1 in]
        n235 = call "Unit Conversion.vi"("환산단위"="N·m", "입력단위"=w797, "입력값"=w798) -> ("환산단위"=w793:string, "환산값 (string)"=w794:string)  [unwired: 3 in, 4 out]
        n236 = Insert Into Array(array=w795, index=5 ("인덱스"), new element #1=w794, new element #2=w793) -> (w791:string[])
      }
      n237 = Index Array(array=w777, index (row) #1=w776, index (row) #2=w782) -> (element #1=w781:string[], element #2=w780:string[])  [unwired: 2 in]
      n238 = Insert Into Array(array=w777, index (row)=w782, new element #1=w780, new element #2=w781, new element #3=w780) -> (w779:string[][])  [unwired: 1 in]
      n239 = Delete From Array(array=w779, length=4 ("길이"), index (col)=w772) -> (deleted portion=w774:string[][], array with subset deleted=w773:string[][])  [unwired: 1 in]
      n240 = Delete From Array(array=w773, length=w772, index (col)=w772) -> (deleted portion=w771:string[][], array with subset deleted=w770:string[][])  [unwired: 1 in]
    }
    frame Default {
      w802 = 3 ("비활성화된 인덱스 (열)")
      n241 = call-poly "Data Classification.vi"("인덱스"=2, "DATA 입력"=w810, "검색 문자열"=w808) -> ("DATA 출력"=w806:string[][])  [unwired: 4 in, 4 out]
      n242 = Delete From Array(array=w806, length=2 ("길이"), index (col)=w802) -> (deleted portion=w804:string[][], array with subset deleted=w803:string[][])  [unwired: 1 in]
      n243 = Delete From Array(array=w803, length=w802, index (col)=w802) -> (deleted portion=w801:string[][], array with subset deleted=w800:string[][])  [unwired: 1 in]
    }
  }
  "Data 2" <- w49
  "Condition" <- w45
  n244 = Equal?(x=w4, y=w2) -> (x = y?=w3:bool)
  n245 = Array Size(array=w45) -> (size(s)=w46:i32[])
  n246 = case shown="참" w3 {
    tunnel: w4 -> [w818 w821]
    tunnel: [w817 w820] -> w1
    tunnel: w2 -> [w816 _]
    frame False {
      n247 = Format Into String(format string="[ %s-%s 교정 ]" ("포맷 문자열"), w818, w816) -> (resulting string=w817:string)  [unwired: 2 in, 1 out]
    }
    frame True {
      n248 = Format Into String(format string="[ %s 교정 ]" ("포맷 문자열"), w821) -> (resulting string=w820:string)  [unwired: 2 in, 1 out]
    }
  }
  "제목" <- w1
  n249 = Index Array(array=w46) -> (element=w47:i32)  [unwired: 1 in]
  n250 = Increment(x=w47) -> (x+1=w48:i32)
  n251 = To Unsigned Long Integer(number=w48) -> (unsigned 32bit integer=w44:u32)
  n252 = property on="제목" class="Str"(reference="제목", error in=w6, "Value"=w1) -> (error out=→"에러 출력":errorcluster)  [unwired: 1 out]
  n253 = Bundle By Name(cluster=T1 {"제목"="", "Condition"=[], "Resolution"=[], "Spec"=[], "Data"=[], "CMC"=[], "NumRows"=0, "Temp_1"=[]} ("클러스터"), "Spec"=w42, "CMC"=w43, "Data"=w49, "Condition"=w45, "Resolution"=w51, "Temp_1"=w14, "NumRows"=w44, "제목"=w1) -> (→"클러스터":T1)
  "Func_ext Out" <- "Func_ext"
